vi "set all channel names.vi"() -> ()   [LabVIEW 2018]
panel:
  in  "Channel Settings File":path=path "C:/Users/User/Documents/Logs/Channel_Settings.csv"
  out "Array":string[](array[string])
  out "concatenated string":string
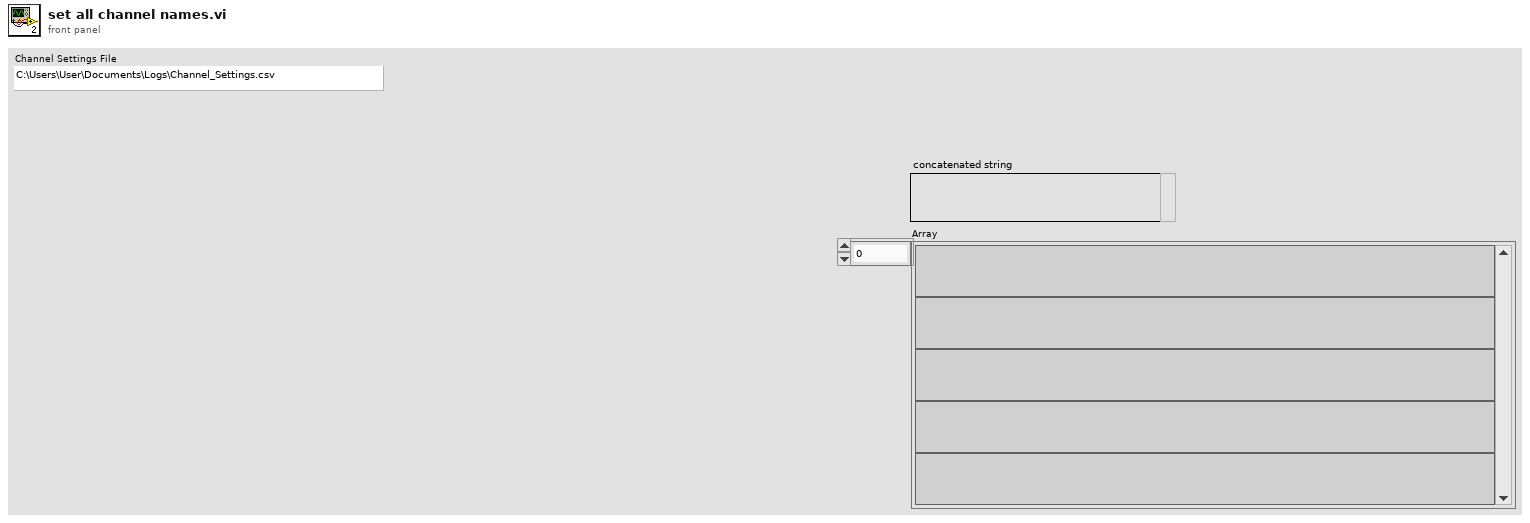
[diagram p1: front panel]
types:
  T1 = typedef "channel_cluster.ctl" = cluster{"Channel Name":string, "Crate":i32, "Card Type":string, "Card":i32, "Channel":i32, "Status Icon":picture, "Vmon (V)":dbl, "Vset (V)":dbl, "Imon (A)":dbl, "Iset (A)":dbl, "Timestamp":string, "ON/OFF":bool, "Status":string, "Vswmax (V)":dbl, "Flag":bool, "Vfile (V)":dbl, "Error Logged":bool[], "enable_file":bool}
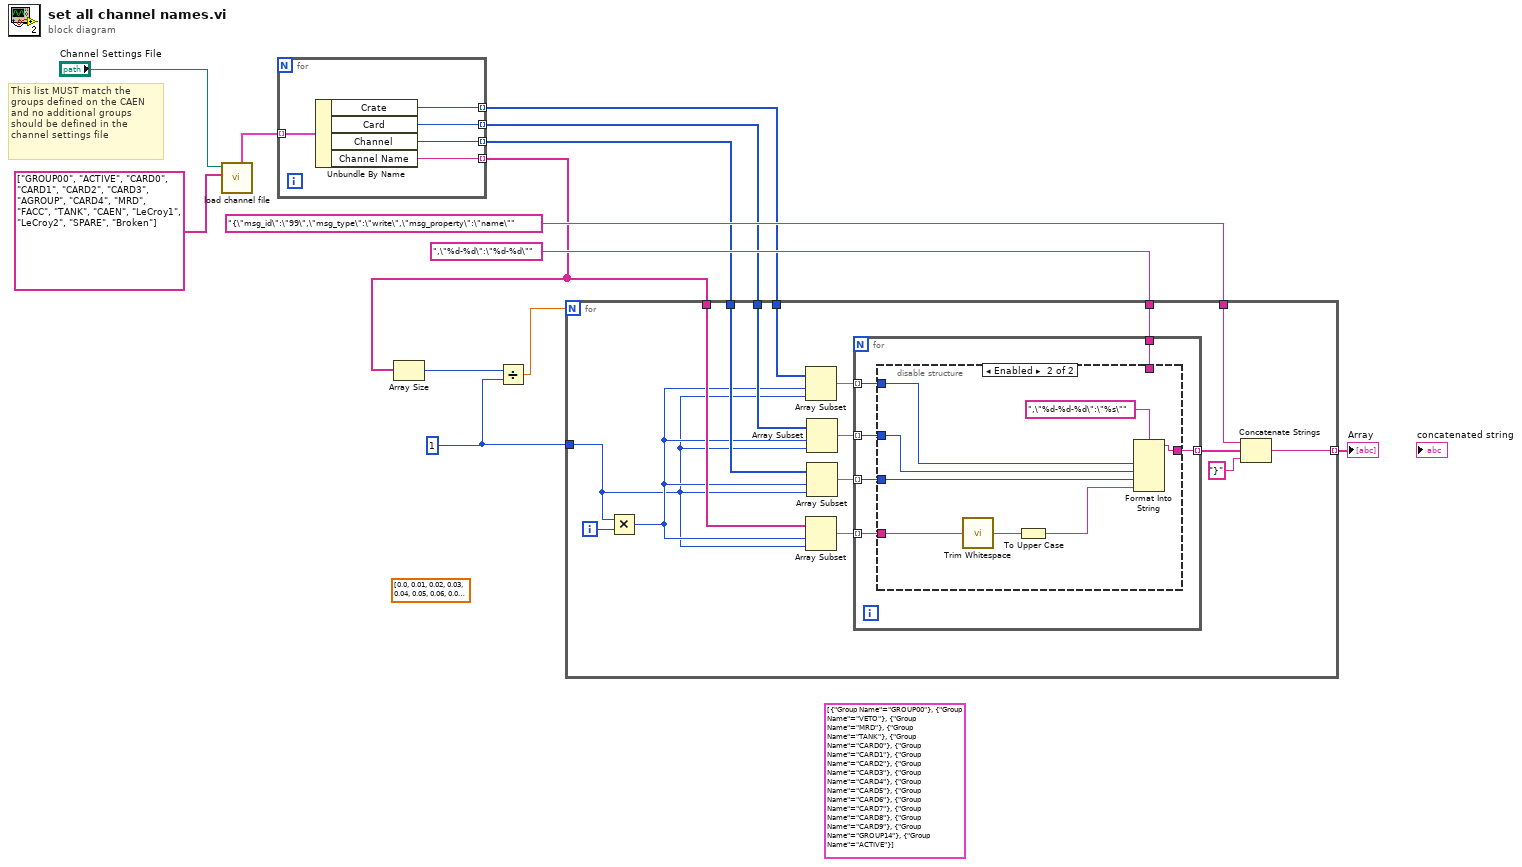
[diagram p0: block diagram]
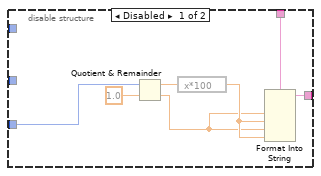
[diagram p2: hidden frame]
diagram:
  (unwired) dbl[] [0.0, 0.01, 0.02, 0.03, 0.04, 0.05, 0.06, 0.07, 0.08, 0.09, 0.1, 0.11, 0.12, 0.13, 0.14, 0.15, 0.16, 0.17, 0.18, 0.19, 0.2, 0.21, 0.22, 0.23, 0.24, 1.0, 1.01, 1.02, 1.03, 1.04, 1.05, 1.06, 1.07, 1.08, 1.09, 1.1, 1.11, 1.12, 1.13, 1.1400000000000001, 1.15, 1.16, 1.17, 1.18, 1.19, 1.2, 1.21, 1.22, 1.23, 1.24, 2.0, 2.01, 2.02, 2.03, 2.04, 2.05, 2.06, 2.07, 2.08, 2.09, 2.1, 2.11, 2.12, 2.13, 2.14, 2.15, 2.16, 2.17, 2.18, 2.19, 2.2, 2.21, 2.22, 2.23, 2.24, 3.0, 3.01, 3.02, 3.03, 3.04, 3.05, 3.06, 3.07, 3.08, 3.09, 3.1, 3.11, 3.12, 3.13, 3.14, 3.15, 3.16, 3.17, 3.18, 3.19, 3.2, 3.21, 3.22, 3.23, 3.24, 4.0, 4.01, 4.02, 4.03, 4.04, 4.05, 4.06, 4.07, 4.08, 4.09, 4.1, 4.11, 4.12, 4.13, 4.14, 4.15, 4.16, 4.17, 4.18, 4.19, 4.2, 4.21, 4.22, 4.23, 4.24, 5.0, 5.01, 5.02, 5.03, 5.04, 5.05, 5.06, 5.07, 5.08, 5.09, 5.1, 5.11, 5.12, 5.13, 5.14, 5.15, 6.0, 6.01, 6.02, 6.03, 6.04, 6.05, 6.06, 6.07, 6.08, 6.09, 6.1, 6.11, 6.12, 6.13, 6.14, 6.15, 7.0, 7.01, 7.02, 7.03, 7.04, 7.05, 7.06, 7.07, 7.08, 7.09, 7.1, 7.11, 7.12, 7.13, 7.14, 7.15, 8.0, 8.01, 8.02, 8.03, 8.04, 8.05, 8.06, 8.07, 8.08, 8.09, 8.1, 8.11, 8.12, 8.13, 8.14, 8.15, 9.0, 9.01, 9.02, 9.03, 9.04, 9.05, 9.06, 9.07, 9.08, 9.09, 9.1, 9.11, 9.12, 9.13, 9.14, 9.15] ("Channels in Group")
  w10 = 1 ("length")
  (unwired) cluster{"Group Name":string}[] [{"Group Name"="GROUP00"}, {"Group Name"="VETO"}, {"Group Name"="MRD"}, {"Group Name"="TANK"}, {"Group Name"="CARD0"}, {"Group Name"="CARD1"}, {"Group Name"="CARD2"}, {"Group Name"="CARD3"}, {"Group Name"="CARD4"}, {"Group Name"="CARD5"}, {"Group Name"="CARD6"}, {"Group Name"="CARD7"}, {"Group Name"="CARD8"}, {"Group Name"="CARD9"}, {"Group Name"="GROUP14"}, {"Group Name"="ACTIVE"}] ("Groups 2")
  # "This list MUST match the\ngroups defined on the CAEN\nand no additional groups\nshould be defined in the \nchannel settings file"
  n1 = call "load channel file.vi"("Group Names"=string[] ["GROUP00", "ACTIVE", "CARD0", "CARD1", "CARD2", "CARD3", "AGROUP", "CARD4", "MRD", "FACC", "TANK", "CAEN", "LeCroy1", "LeCroy2", "SPARE", "Broken"], "Channel List"="Channel Settings File") -> ("Array"=w6:T1[])  [unwired: 5 in, 4 out]
  n2 = for {
    tunnel: w6 -> [w18] mode=indexing
    tunnel: [w17] -> w5 mode=indexing
    tunnel: [w16] -> w4 mode=indexing
    tunnel: [w15] -> w3 mode=indexing
    tunnel: [w14] -> w2 mode=indexing
    n3 = Unbundle By Name(w18) -> ("Crate"=w14:i32, "Card"=w15:i32, "Channel"=w16:i32, "Channel Name"=w17:string)
  }
  n4 = Array Size(array=w5) -> (size(s)=w1:i32)
  n5 = Divide(x=w1, y=w10) -> (x/y=w9:dbl)
  n6 = for {
    N: w9 -> [_]
    tunnel: ",\"%d-%d\":\"%d-%d\"" ("format string") -> [w34]
    tunnel: w5 -> [w25]
    tunnel: "{\"msg_id\":\"99\",\"msg_type\":\"write\",\"msg_property\":\"name\"" ("format string") -> [w30]
    tunnel: [w31] -> w11 mode=indexing
    tunnel: w10 -> [w20]
    tunnel: w4 -> [w26]
    tunnel: w3 -> [w24]
    tunnel: w2 -> [w22]
    i -> [w29]
    n7 = Multiply(x=w20, y=w29) -> (x*y=w21:i32)
    n8 = Array Subset(array=w22, index=w21, length=w20) -> (w19:i32[])
    n9 = Array Subset(array=w25, index=w21, length=w20) -> (w27:string[])
    n10 = Array Subset(array=w24, index=w21, length=w20) -> (w23:i32[])
    n11 = Array Subset(array=w26, index=w21, length=w20) -> (w28:i32[])
    n12 = for {
      tunnel: w28 -> [w40] mode=indexing
      tunnel: w34 -> [w39]
      tunnel: [w38] -> w33 mode=indexing
      tunnel: w27 -> [w37] mode=indexing
      tunnel: w23 -> [w36] mode=indexing
      tunnel: w19 -> [w35] mode=indexing
      n13 = disable-structure shown="Enabled" {
        disable-tunnel: w40 -> [w47 w50]
        disable-tunnel: w39 -> [w44 _]
        disable-tunnel: [w43 w55] -> w38
        disable-tunnel: w37 -> [_ w51]
        disable-tunnel: w36 -> [_ w49]
        disable-tunnel: w35 -> [_ w48]
        frame Disabled {
          n14 = Quotient & Remainder(x=w47, y=1.0) -> (x-y*floor(x/y)=w45:dbl, floor(x/y)=w41:dbl)
          n15 = expression code="x*100"(w45) -> (w42:dbl)
          n16 = Format Into String(format string=w44, w41, w42, w41, w42) -> (resulting string=w43:string)  [unwired: 2 in, 1 out]
        }
        frame Enabled {
          n17 = call <vilib>:"Trim Whitespace.vi"("string"=w51) -> ("trimmed string"=w53:string)  [unwired: 1 in]
          n18 = To Upper Case(1:w53) -> (0:w52:string)
          n19 = Format Into String(format string=",\"%d-%d-%d\":\"%s\"", w48, w49, w50, w52) -> (resulting string=w55:string)  [unwired: 2 in, 1 out]
        }
      }
    }
    n20 = Concatenate Strings(w30, w33, "}" ("string")) -> (w31:string)
  }
  "Array" <- w11
